vi "AM DSB.vi"() -> ()   [LabVIEW 2018]
uses:
  <vilib>/measure/maspectr.llb/FFT Spectrum (Mag-Phase) for N Chan.vi
  <vilib>/measure/NI_MAPro.lvlib
panel:
  in  "stop":bool
  in  "Tab Control":enum32{"Tempo", "Frequência"}(tab)
  out "Tempo Modulada":dynamicdata(graph)
  out "Tempo Infomação":dynamicdata(graph)
  out "Tempo Portadora":dynamicdata(graph)
  out "Frequência Modulada":cluster{"f0":dbl, "df":dbl, "magnitude":dbl[]}[](graph)
  out "Frequência Informação":cluster{"f0":dbl, "df":dbl, "magnitude":dbl[]}[](graph)
  out "Frequência Portadora":cluster{"f0":dbl, "df":dbl, "real part":dbl[]}[](graph)
  in  "Frequência Informação":dbl(slide) scale=0.0..50.0
  in  "Amplitude Informação":dbl(slide) scale=0.0..10.0
  in  "Frequência Portadora":dbl(slide) scale=0.0..750.0
  in  "Amplitude Portadora":dbl(slide) scale=0.0..10.0
  in  "Offset DC":dbl(slide) scale=0.0..10.0
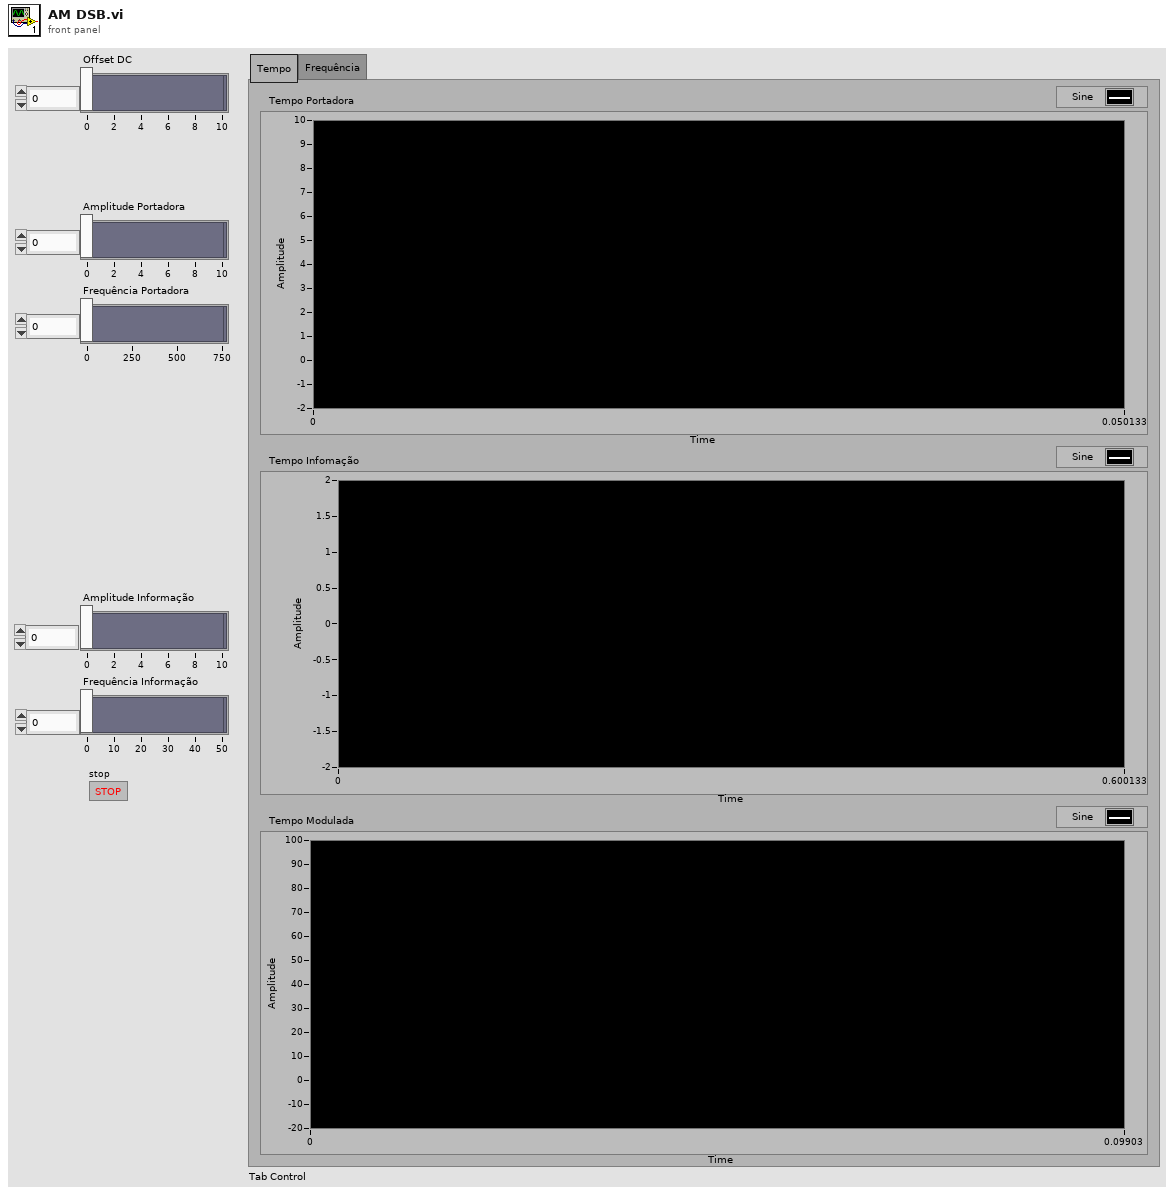
[diagram p1: front panel]
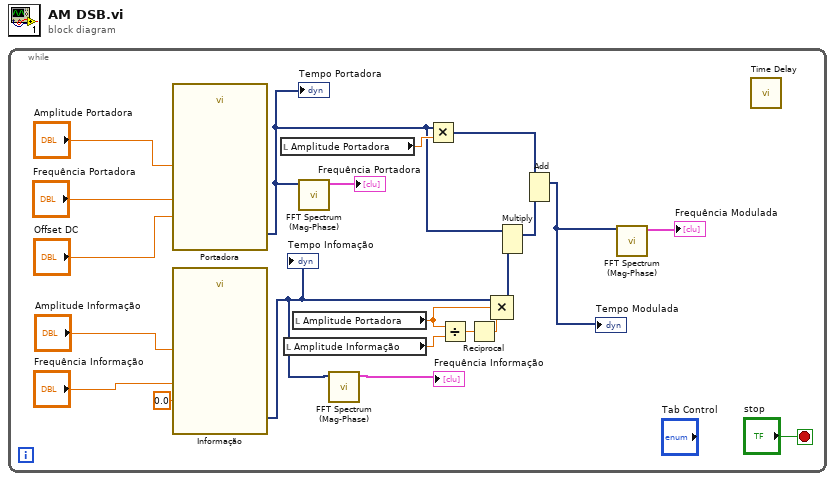
[diagram p0: block diagram]
diagram:
  n1 = while {
    stop <- "stop" stop-if-true
    n2 = call "Portadora"("Offset"="Offset DC", "Frequency"="Frequência Portadora", "Amplitude"="Amplitude Portadora") -> ("Sine"=w8:dynamicdata)  [unwired: 11 in, 1 out]
    "Tempo Portadora" <- w8
    n3 = call "Informação"("Offset"=0.0, "Frequency"="Frequência Informação", "Amplitude"="Amplitude Informação") -> ("Sine"=w6:dynamicdata)  [unwired: 11 in, 1 out]
    "Tempo Infomação" <- w6
    n4 = local read "Amplitude Portadora"() -> (w15:dbl)
    n5 = local read "Amplitude Informação"() -> (w2:dbl)
    n6 = local read "Amplitude Portadora"() -> (w1:dbl)
    n7 = call-poly <vilib>:"FFT Spectrum (Mag-Phase).vi"("time signals"=w8) -> ("magnitudes"=→"Frequência Portadora":cluster{"f0":dbl, "df":dbl, "magnitude":dbl[]}[])  [unwired: 6 in, 4 out]
    n8 = call-poly <vilib>:"FFT Spectrum (Mag-Phase).vi"("time signals"=w6) -> ("magnitudes"=→"Frequência Informação":cluster{"f0":dbl, "df":dbl, "magnitude":dbl[]}[])  [unwired: 6 in, 4 out]
    n9 = Multiply(x=w8, y=w15) -> (x*y=w11:dynamicdata)
    n10 = Divide(x=w1, y=w2) -> (x/y=w14:dbl)
    n11 = Reciprocal(x=w14) -> (1/x=w13:dbl)
    n12 = Compound Arithmetic op=MULTIPLY(w6, w1, w13) -> (w12:dynamicdata)
    n13 = Multiply(1:w12, 2:w8) -> (0:w10:dynamicdata)  [unwired: 1 in, 1 out]
    n14 = Add(1:w10, 2:w11) -> (0:w3:dynamicdata)  [unwired: 1 in, 1 out]
    "Tempo Modulada" <- w3
    n15 = call-poly <vilib>:"FFT Spectrum (Mag-Phase).vi"("time signals"=w3) -> ("magnitudes"=→"Frequência Modulada":cluster{"f0":dbl, "df":dbl, "magnitude":dbl[]}[])  [unwired: 6 in, 4 out]
    n16 = call "Time Delay"() -> ()  [unwired: 11 in, 1 out]
  }
